vi "field_sweep.vi"() -> ()   [LabVIEW 2017]
uses:
  Controls/State.ctl
  Controls/Data.ctl
  <vilib>/Utility/error.llb/DialogType.ctl
  <vilib>/DAQmx/write.llb/DAQmx Write (Analog DBL 1Chan 1Samp).vi
  <vilib>/DAQmx/create/channels.llb/DAQmx Create Channel (AO-Voltage-Basic).vi
  <vilib>/DAQmx/miscellaneous.llb/DAQmx Fill In Error Info.vi
  <instrlib>/niVNA/niVNA.llb/niVNA Fetch Sweep Measurement (DBL).vi
  <instrlib>/LakeShore 336/Public/Data/Sensor Data (Single Reading).vi
  <instrlib>/LakeShore 336/Lake Shore 336.lvlib
panel:
  in  "Folder":path caption="Folder for saving"
  out "Temp. Cont. Name (out)":refnum<visa-resource-name>
  in  "Temp. Cont. Name (in)":refnum<visa-resource-name>
  in  "Auto Save flag":bool
  out "Gaussmeter Name (out)":refnum<visa-resource-name>="Lakeshore_475"
  in  "Gaussmeter Name (in)":refnum<visa-resource-name>="Lakeshore_475"
  in  "Clear button":bool
  in  "Hysteresis":bool caption="Hysteresis On/Off"
  out "DAQ channel (out)":tag="DAQ_6363/ao1"
  in  "Averaging Points":i32=10 min=1 max=3201 step=1
  in  "DAQ channel (in)":tag="DAQ_6363/ao1"
  in  "Exit Button":bool
  in  "IF Bandwidth":dbl(ring)=1000.0 items=["10 Hz"=10.0, "30 Hz"=30.0, "100 Hz"=100.0, "300 Hz"=300.0, "1 KHz"=1000.0, "3 KHz"=3000.0, "10 KHz"=10000.0, "30 KHz"=30000.0]
  in  "Speed (Oe/sec)":dbl=50.0
  in  "Frequency (Hz)":dbl=3000000000.0 min=10000000.0 max=6000000000.0
  in  "Save Button":bool
  out "Status":string="Off"
  out "Cursor":cluster{"x":dbl, "y":dbl} {"x" format="%.2f"; "y" format="%.5f"}
  out "VNA Name (out)":refnum<k15>="VNA_5630"
  out "Error (out)":errorcluster
  in  "Error (in) (no error)":errorcluster
  in  "Format":i32(ring)=1 items=["Log Magnitude (dB)"=0, "Lin Magnitude"=1, "Phase (deg)"=2, "VSWR"=3, "Group Delay"=6]
  out "SpectrumGraph":cluster{"Old Field":dbl[], "Old Signal":dbl[]}[](graph)
  in  "S-parameter":i32(ring)=1 caption="Measurement" items=["S11", "S21"]
  in  "Start Button":bool
  in  "Stop Button":bool
  in  "Output Power (dBm)":dbl=1.0 min=-25.0 max=5.0 step=0.5
  in  "Number of Points":i32=1000 min=1 max=3201 step=1
  in  "Stop H Field (Oe)":dbl=1500.0 min=-6000.0 max=6000.0 format="%#_6f"
  in  "Start H Field (Oe)":dbl=1000.0 min=-6000.0 max=6000.0 format="%#_6f"
  in  "VNA Name (in)":refnum<k15>="VNA_5630"
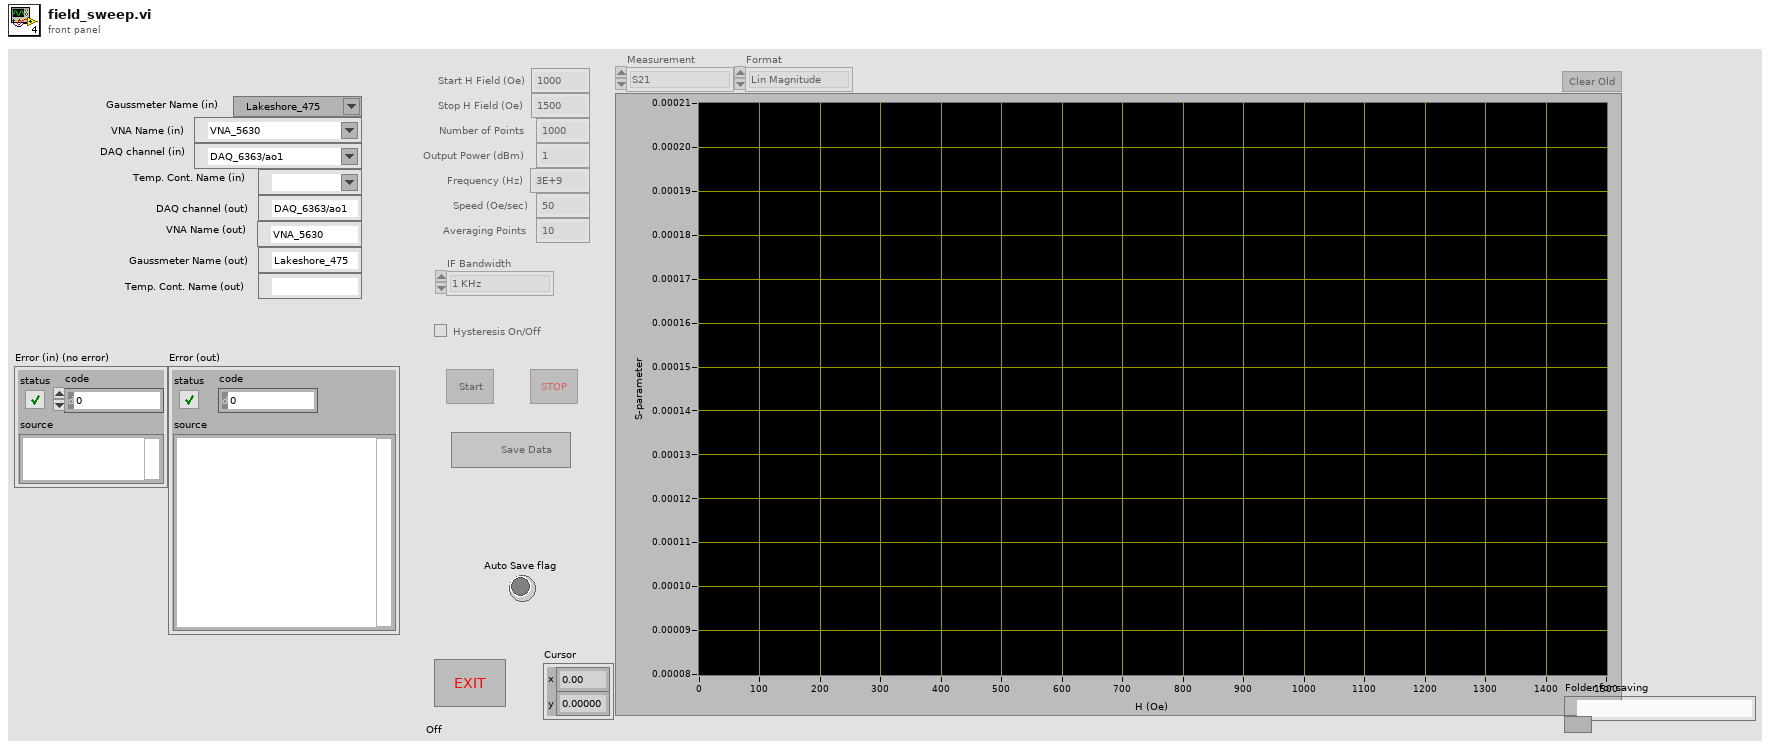
[diagram p1: front panel]
types:
  T1 = cluster{"DAQ task":refnum<k21>, "DAQ channel":tag, "VNA Name":refnum<k15>, "Gaussmeter Name":refnum<visa-resource-name>, "Temp. Cont. Name":refnum<visa-resource-name>}
  T2 = typedef "Data.ctl" = cluster{"Field":dbl[], "Signal":dbl[], "Temperature":dbl[], "Old Field":dbl[], "Old Signal":dbl[], "Old Temperature":dbl[]}
  T3 = typedef "State.ctl" = enum16{"Init", "Idle", "Sweeping up", "Sweeping down", "Running", "Running down", "Shutdown"}
  T4 = cluster{"Baud Rate":u32, "Parity":u16, "Data Bits":u16, "Stop Bits":u16, "Flow Control":u16}
  T5 = typedef "DialogType.ctl" = u16
  T6 = typedef "LVPoint32TypeDef.ctl" = cluster{"Horizontal":i32, "Vertical":i32}
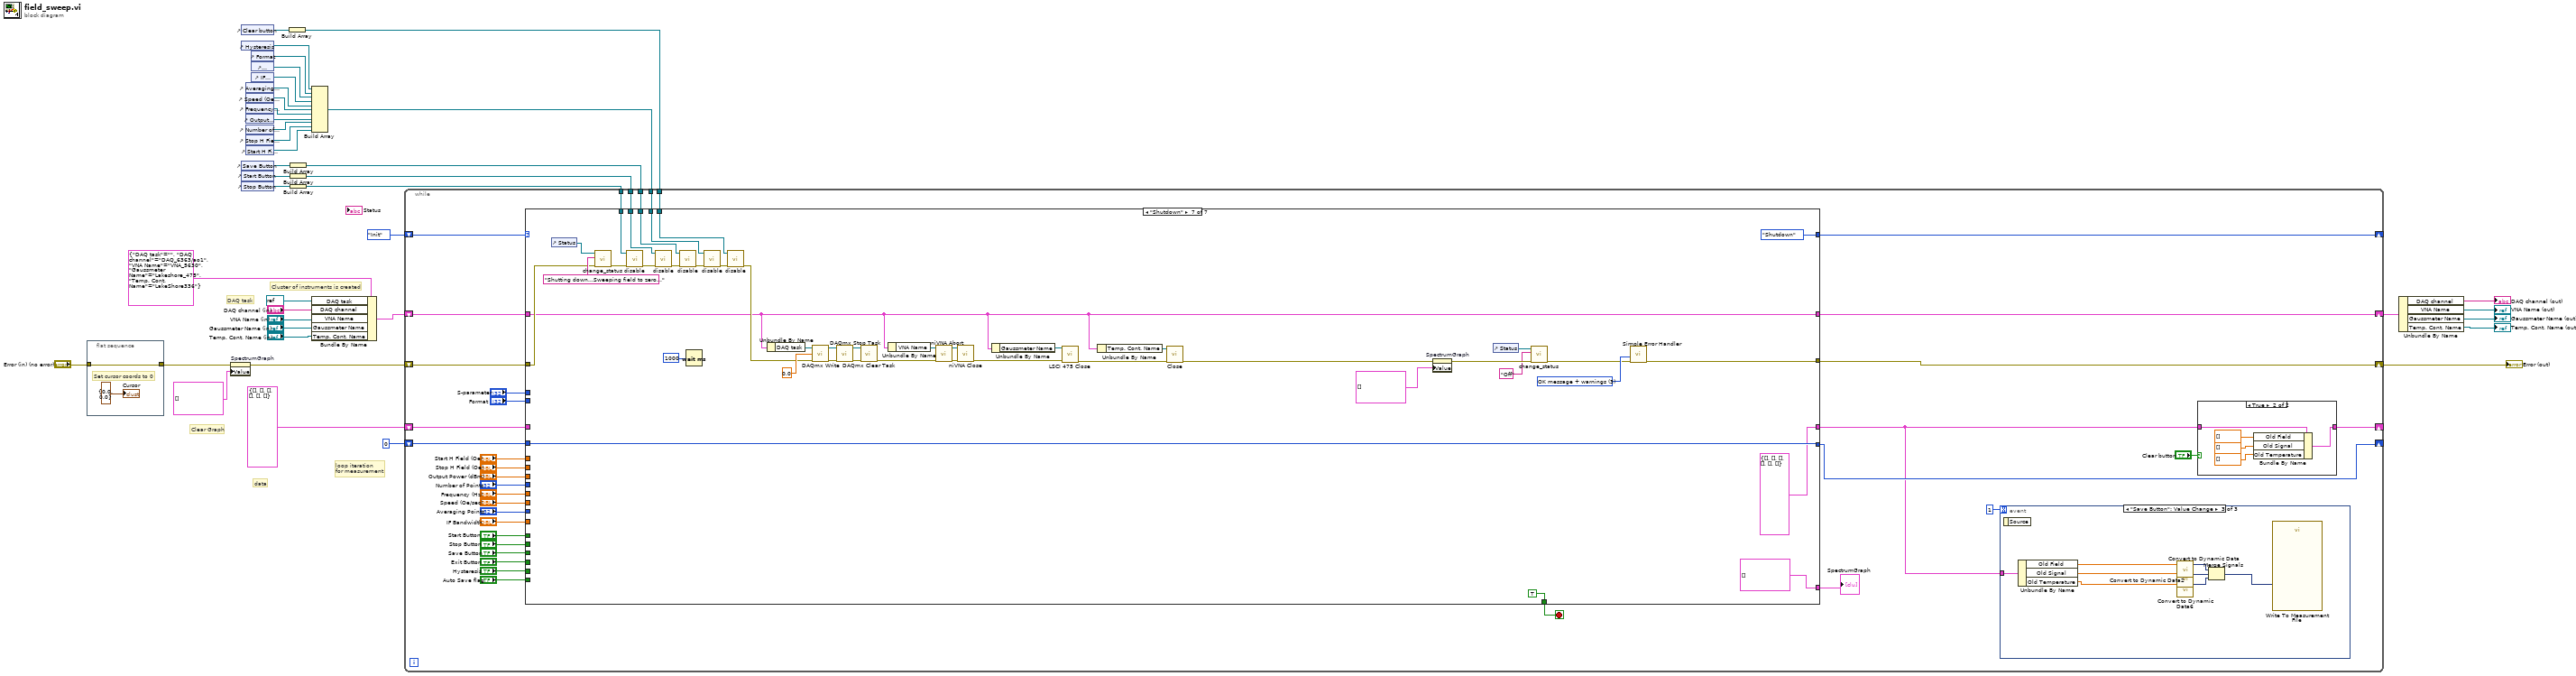
[diagram p0: block diagram]
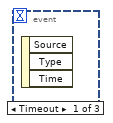
[diagram p3: hidden frame]
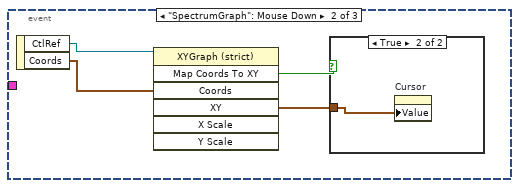
[diagram p4: hidden frame]
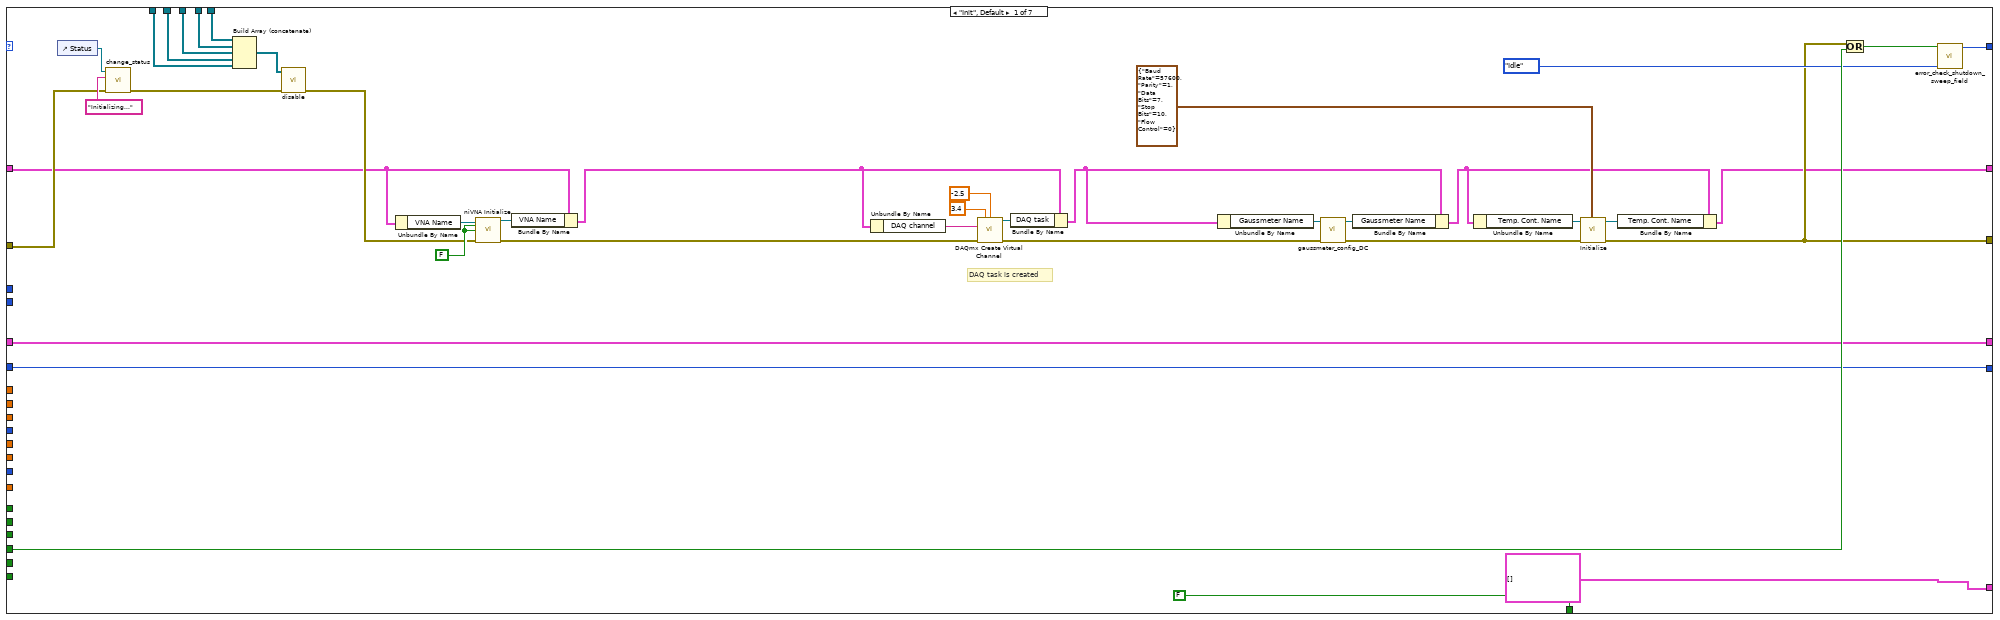
[diagram p6: hidden frame]
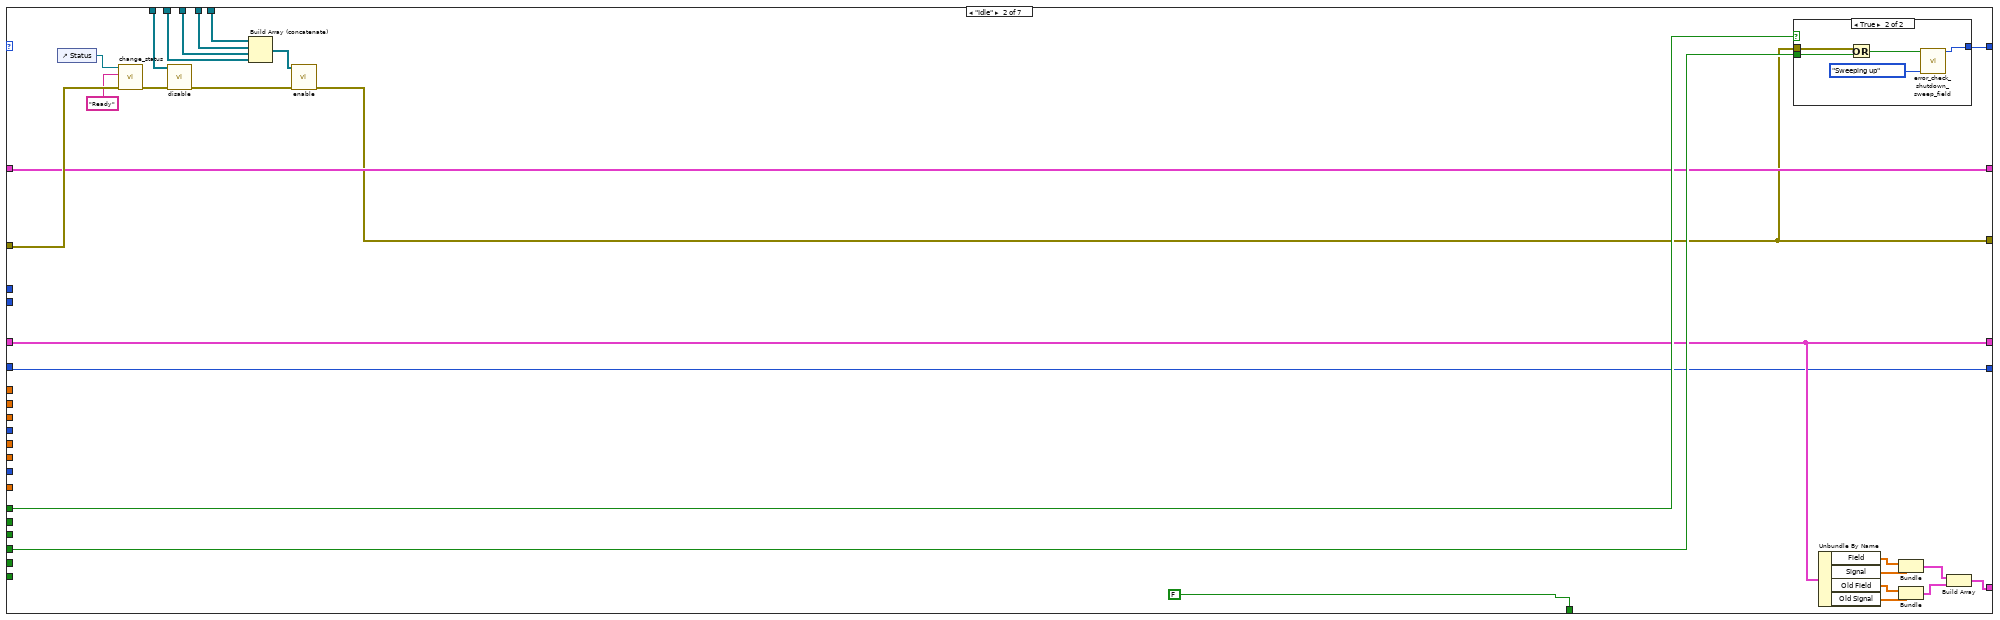
[diagram p7: hidden frame]
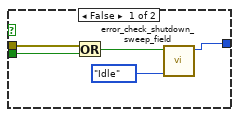
[diagram p8: hidden frame]
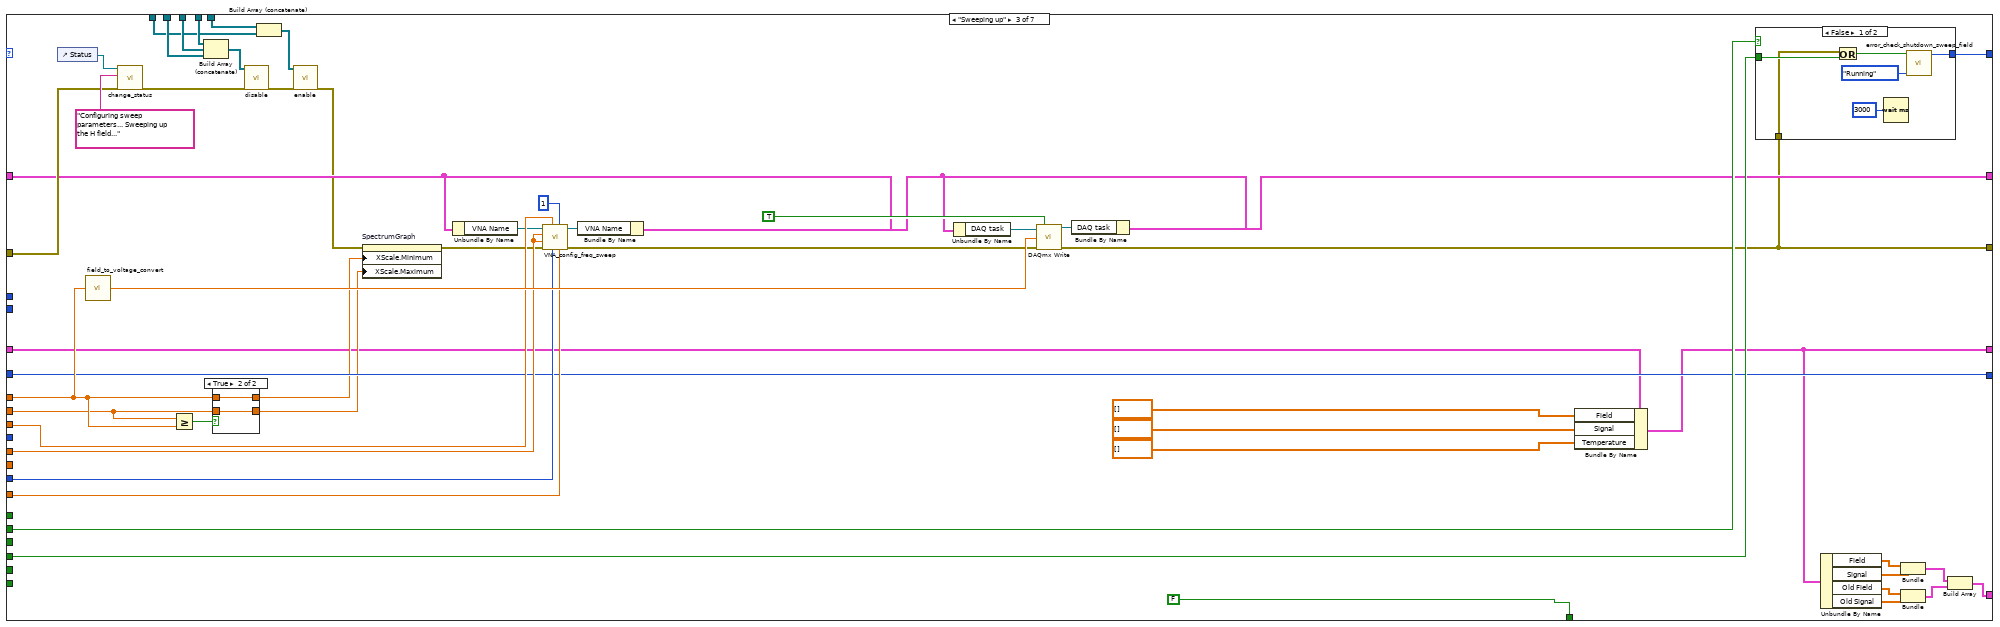
[diagram p9: hidden frame]
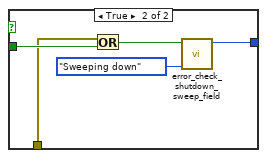
[diagram p11: hidden frame]
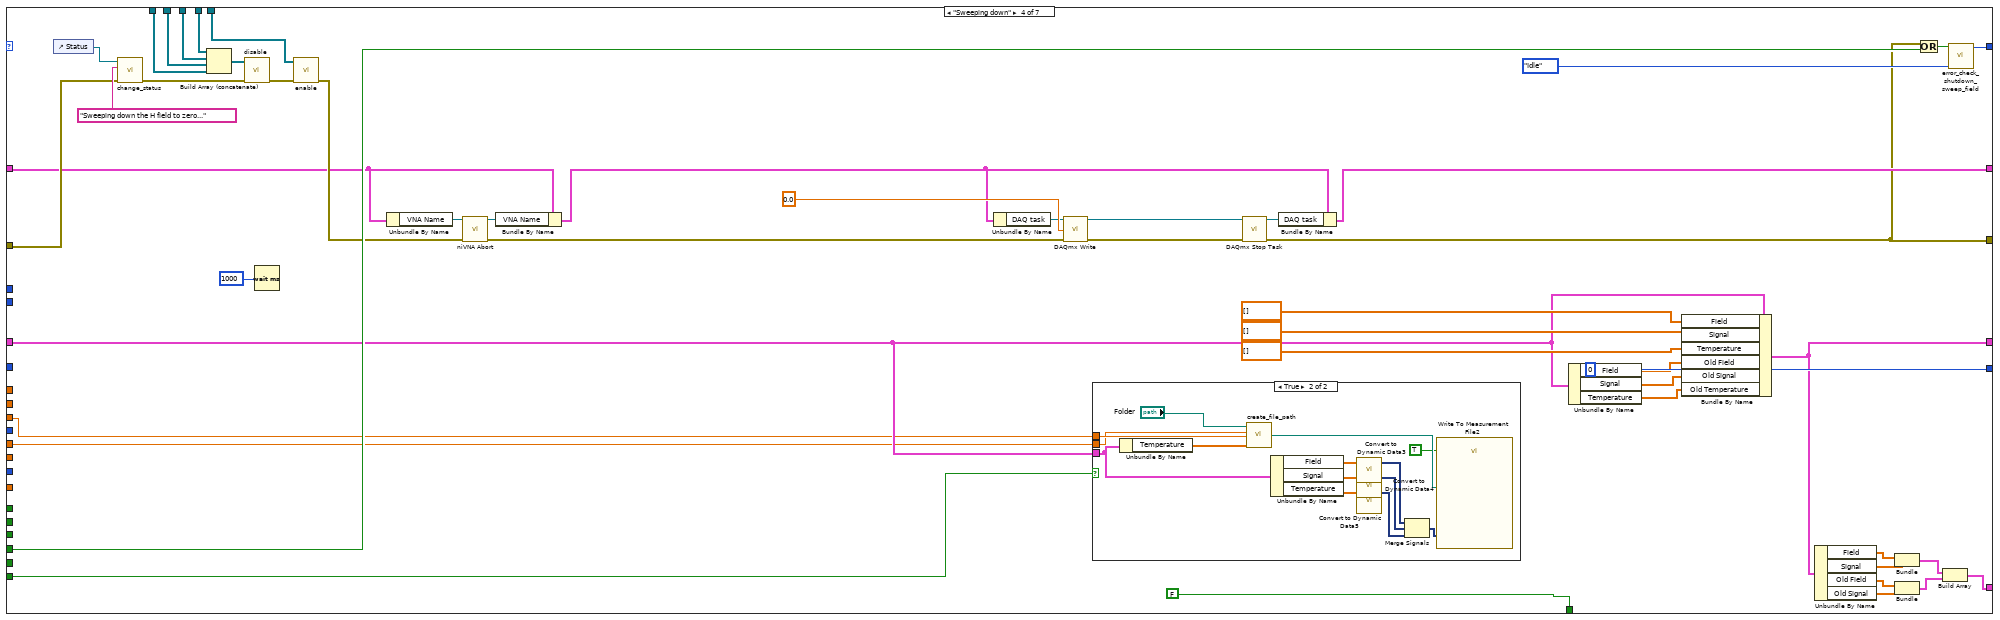
[diagram p12: hidden frame]
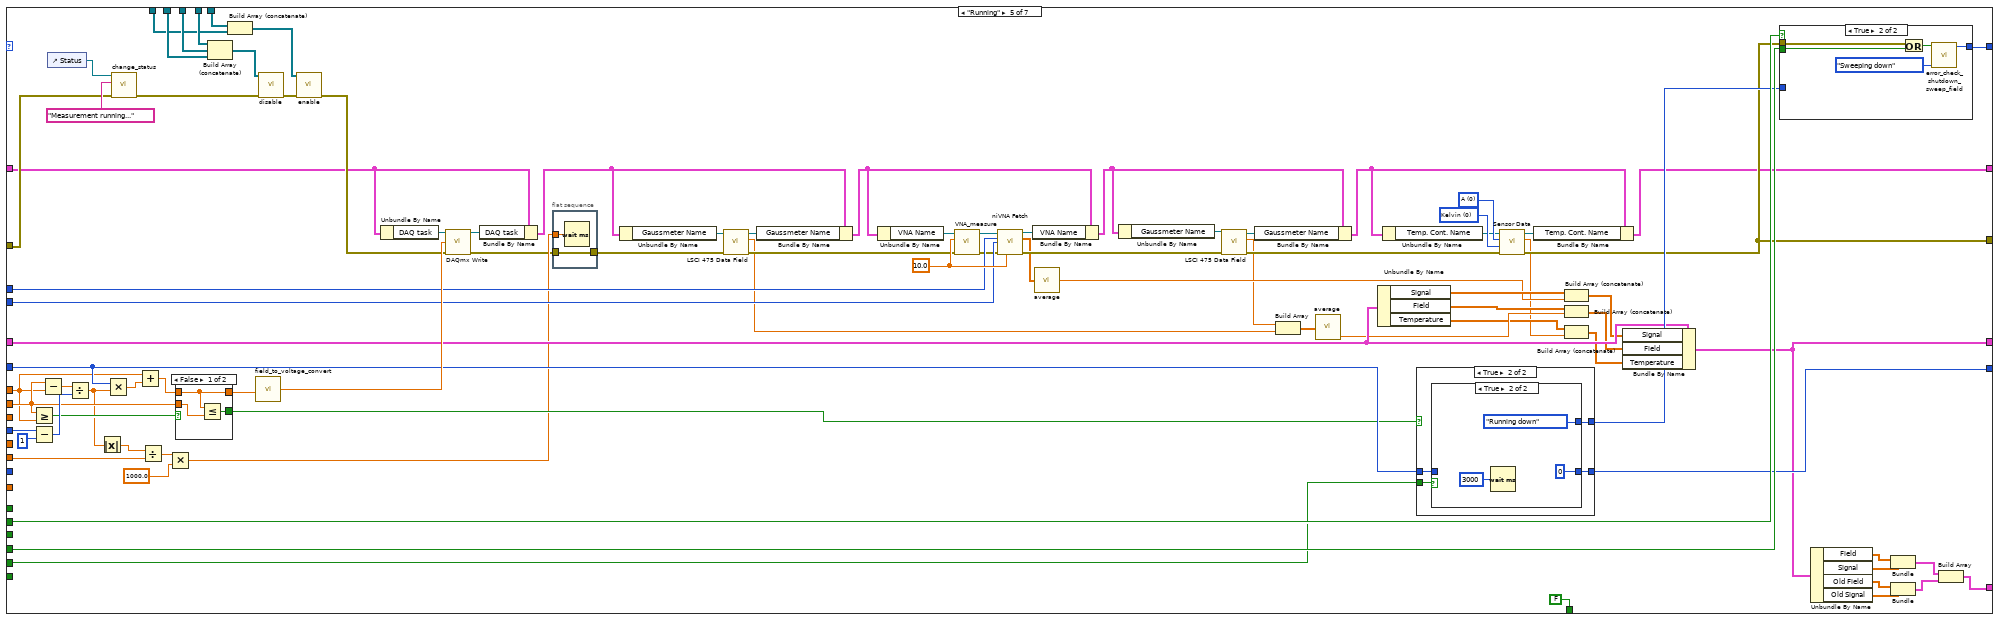
[diagram p14: hidden frame]
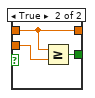
[diagram p15: hidden frame]
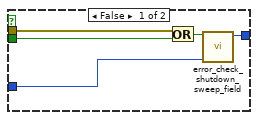
[diagram p16: hidden frame]
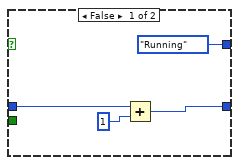
[diagram p17: hidden frame]
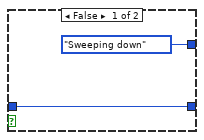
[diagram p18: hidden frame]
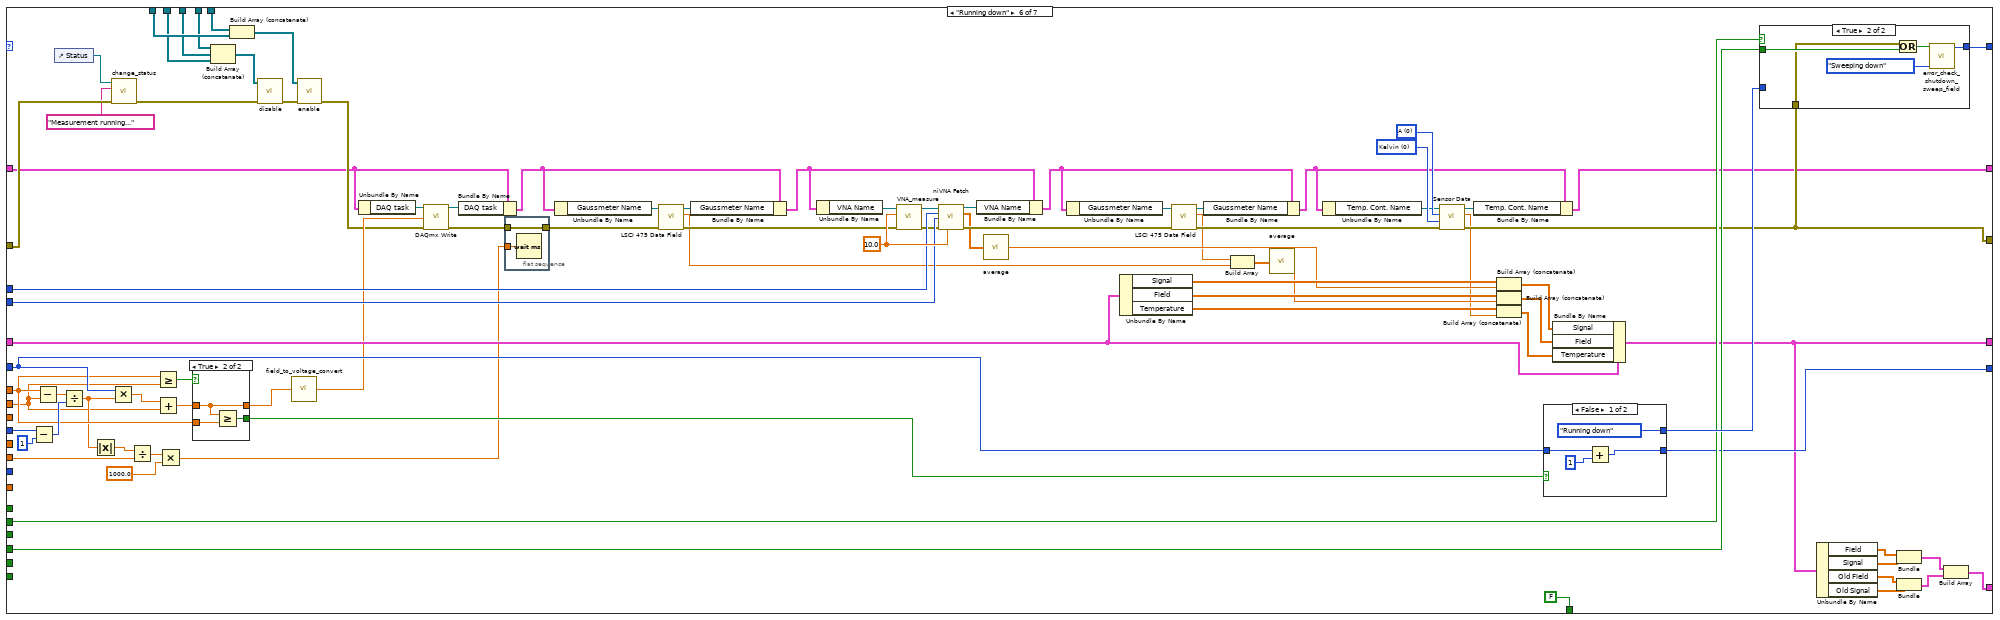
[diagram p19: hidden frame]
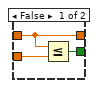
[diagram p20: hidden frame]
diagram:
  # "data"
  # "Cluster of instruments is created"
  # "loop iteration\nfor measurement"
  # "DAQ task"
  # "Clear Graph"
  n1 = flat-sequence {
    tunnel: "Error (in) (no error)" -> [w41]
    tunnel: [w41] -> w7
    frame #0 {
      # "Set cursor coords to 0"
      "Cursor" <- cluster{"x":dbl, "y":dbl} {"x"=0.0, "y"=0.0} ("Cursor")
    }
  }
  n2 = property on="SpectrumGraph" class="XYGraph (strict)"(error in=w7, "Value"=cluster{"Old Field":dbl[], "Old Signal":dbl[]}[] [] ("SpectrumGraph")) -> (error out=w23:errorcluster)  [unwired: 1 in, 1 out]
  n3 = control-ref of="Clear button"() -> (w16:refnum<vi>)
  n4 = control-ref of="Hysteresis"() -> (w17:refnum<vi>)
  n5 = control-ref of="Save Button"() -> (w27:refnum<vi>)
  n6 = control-ref of="Start Button"() -> (w32:refnum<vi>)
  n7 = control-ref of="Stop Button"() -> (w31:refnum<vi>)
  n8 = control-ref of="Averaging Points"() -> (w24:refnum<vi>)
  n9 = control-ref of="Speed (Oe/sec)"() -> (w38:refnum<vi>)
  n10 = control-ref of="Frequency (Hz)"() -> (w37:refnum<vi>)
  n11 = control-ref of="Output Power (dBm)"() -> (w36:refnum<vi>)
  n12 = control-ref of="Number of Points"() -> (w35:refnum<vi>)
  n13 = control-ref of="Stop H Field (Oe)"() -> (w34:refnum<vi>)
  n14 = control-ref of="Start H Field (Oe)"() -> (w33:refnum<vi>)
  n15 = control-ref of="Format"() -> (w18:refnum<vi>)
  n16 = control-ref of="S-parameter"() -> (w19:refnum<vi>)
  n17 = control-ref of="IF Bandwidth"() -> (w39:refnum<vi>)
  n18 = Build Array(w16) -> (w15:refnum<vi>[])
  n19 = Build Array(w27) -> (w26:refnum<vi>[])
  n20 = Build Array(w32) -> (w29:refnum<vi>[])
  n21 = Build Array(w31) -> (w28:refnum<vi>[])
  n22 = Bundle By Name(cluster=T1 {"DAQ task"="", "DAQ channel"="DAQ_6363/ao1", "VNA Name"="VNA_5630", "Gaussmeter Name"="Lakeshore_475", "Temp. Cont. Name"="LakeShore336"} ("Cluster"), "DAQ task"=refnum<k21> refnum ("task in"), "DAQ channel"="DAQ channel (in)", "VNA Name"="VNA Name (in)", "Gaussmeter Name"="Gaussmeter Name (in)", "Temp. Cont. Name"="Temp. Cont. Name (in)") -> (w9:T1)
  n23 = Build Array(w17, w18, w19, w39, w24, w38, w37, w36, w35, w34, w33) -> (w30:refnum<vi>[])
  n24 = while {
    shift-right: [w74] -> _
    shift-left: State."Init" -> [w78]
    shift-right: [w57] -> _
    shift-left: 0 -> [w59]
    tunnel: w30 -> [w77]
    tunnel: w29 -> [w76]
    tunnel: w28 -> [w75]
    shift-right: [w73] -> w20
    shift-left: w23 -> [w72]
    tunnel: w26 -> [w71]
    shift-right: [w48] -> _
    shift-left: T2 {"Field"=[], "Signal"=[], "Temperature"=[], "Old Field"=[], "Old Signal"=[], "Old Temperature"=[]} ("Cluster") -> [w54]
    tunnel: w15 -> [w47]
    shift-right: [w45] -> w6
    shift-left: w9 -> [w46]
    stop <- w66 stop-if-true
    n25 = case shown="\"Shutdown\"" w78 {
      tunnel: w77 -> [w103 w142 w184 w260 w311 w429 w571]
      tunnel: w76 -> [w101 w140 w182 w258 w309 w427 w573]
      tunnel: w75 -> [w100 w163 w179 w257 w306 w430 w574]
      tunnel: w72 -> [w134 w161 w223 w288 w391 w513 w569]
      tunnel: [w129 w157 w220 w284 w376 w493 State."Shutdown"] -> w74
      tunnel: [w110 w144 w189 w261 w322 w441 w544] -> w73
      tunnel: w71 -> [w102 w141 w183 w259 w310 w428 w572]
      tunnel: "Start Button" -> [_ w158 _ _ _ _ _]
      tunnel: "Stop Button" -> [_ _ w222 _ w379 w501 _]
      tunnel: "Save Button" -> [_ _ _ _ _ _ _]
      tunnel: "Exit Button" -> [w130 w156 w219 w285 w378 w494 _]
      tunnel: [FALSE FALSE FALSE FALSE FALSE FALSE TRUE] -> w66
      tunnel: "Start H Field (Oe)" -> [_ _ w210 _ w352 w484 _]
      tunnel: "Stop H Field (Oe)" -> [_ _ w209 _ w364 w472 _]
      tunnel: "Output Power (dBm)" -> [_ _ w217 w242 _ _ _]
      tunnel: "Number of Points" -> [_ _ _ _ w386 w487 _]
      tunnel: "Frequency (Hz)" -> [_ _ w218 w243 _ _ _]
      tunnel: "Speed (Oe/sec)" -> [_ _ _ _ w387 w477 _]
      tunnel: w59 -> [w127 w146 w201 _ w380 w488 w559]
      tunnel: "Averaging Points" -> [_ _ w216 _ _ _ _]
      tunnel: [w127 w146 w201 0 w349 w470 w559] -> w57
      tunnel: "IF Bandwidth" -> [_ _ w214 _ _ _ _]
      tunnel: [w125 w147 w185 w268 w348 w469 T2 {"Field"=[], "Signal"=[], "Temperature"=[], "Old Field"=[], "Old Signal"=[], "Old Temperature"=[]} ("Cluster")] -> w43
      tunnel: w54 -> [w125 w147 w186 w244 w374 w500 _]
      tunnel: "Hysteresis" -> [_ _ _ _ w362 _ _]
      tunnel: "S-parameter" -> [_ _ _ _ w361 w503 _]
      tunnel: "Format" -> [_ _ _ _ w360 w502 _]
      tunnel: [cluster{"Old Field":dbl[], "Old Signal":dbl[]}[] [] w148 w202 w269 w359 w483 cluster{"Old Field":dbl[], "Old Signal":dbl[]}[] []] -> w50
      tunnel: w47 -> [w104 w143 w181 w266 w307 w431 w550]
      tunnel: w46 -> [w118 w145 w198 w250 w344 w465 w539]
      tunnel: [w105 w145 w190 w264 w319 w439 w539] -> w45
      tunnel: "Auto Save flag" -> [_ _ _ w241 _ _ _]
      frame "Init", Default {
        w135 = FALSE ("id query")
        # "DAQ task is created"
        n26 = control-ref of="Status"() -> (w137:refnum<vi>)
        n27 = call "change_status.vi"("error in (no error)"=w134, "String"="Initializing...", "String in"=w137) -> ("error out"=w98:errorcluster)  [unwired: 8 in]
        n28 = Build Array (concatenate)(w104, w103, w102, w101, w100) -> (w99:refnum<vi>[])
        n29 = call "disable.vi"("error in (no error)"=w98, "Array"=w99) -> ("error out"=w122:errorcluster)  [unwired: 9 in]
        n30 = Unbundle By Name(w118) -> ("VNA Name"=w121:refnum<k15>)
        n31 = call <instrlib>:"niVNA Initialize.vi"("resource name"=w121, "id query"=w135, "reset"=w135, "error in"=w122) -> ("instrument handle"=w116:refnum<k15>, "error out"=w133:errorcluster)  [unwired: 10 in]
        n32 = Bundle By Name(cluster=w118, "VNA Name"=w116) -> (w117:T1)
        n33 = Unbundle By Name(w117) -> ("DAQ channel"=w120:tag)
        n34 = call-poly <vilib>:"DAQmx Create Virtual Channel.vi"("maximum value"=3.4, "minimum value"=-2.5, "physical channels"=w120, "error in"=w133) -> ("task out"=w119:refnum<k21>, "error out"=w115:errorcluster)  [unwired: 10 in]
        n35 = Bundle By Name(cluster=w117, "DAQ task"=w119) -> (w112:T1)
        n36 = Unbundle By Name(w112) -> ("Gaussmeter Name"=w114:refnum<visa-resource-name>)
        n37 = call "gaussmeter_config_DC.vi"("error in (no error)"=w115, "VISA Refnum in"=w114) -> ("error out"=w111:errorcluster, "VISA Refnum out"=w113:refnum<visa-resource-name>)  [unwired: 8 in]
        n38 = Bundle By Name(cluster=w112, "Gaussmeter Name"=w113) -> (w106:T1)
        n39 = Unbundle By Name(w106) -> ("Temp. Cont. Name"=w108:refnum<visa-resource-name>)
        n40 = call <instrlib>:"Initialize.vi"("Serial Configuration"=T4 {"Baud Rate"=57600, "Parity"=1, "Data Bits"=7, "Stop Bits"=10, "Flow Control"=0}, "error in (no error)"=w111, "VISA resource name"=w108) -> ("error out"=w110:errorcluster, "VISA resource name out"=w107:refnum<visa-resource-name>)  [unwired: 7 in]
        n41 = Bundle By Name(cluster=w106, "Temp. Cont. Name"=w107) -> (w105:T1)
        n42 = Or(x=w110, y=w130) -> (x .or. y?=w128:bool)
        n43 = call "error_check_shutdown_sweep_field.vi"("State In"=State."Idle", "Boolean"=w128) -> ("State Out"=w129:T3)  [unwired: 9 in]
      }
      frame "Idle" {
        n44 = control-ref of="Status"() -> (w160:refnum<vi>)
        n45 = call "change_status.vi"("error in (no error)"=w161, "String"="Ready", "String in"=w160) -> ("error out"=w162:errorcluster)  [unwired: 8 in]
        n46 = call "disable.vi"("error in (no error)"=w162, "Array"=w163) -> ("error out"=w138:errorcluster)  [unwired: 9 in]
        n47 = Build Array (concatenate)(w143, w142, w141, w140) -> (w139:refnum<vi>[])
        n48 = call "enable.vi"("error in (no error)"=w138, "Array"=w139) -> ("error out"=w144:errorcluster)  [unwired: 9 in]
        n49 = case shown="True" w158 {
          tunnel: [w167 w171] -> w157
          tunnel: w156 -> [w166 w172]
          tunnel: w144 -> [w164 w169]
          frame False {
            n50 = Or(x=w164, y=w166) -> (x .or. y?=w168:bool)
            n51 = call "error_check_shutdown_sweep_field.vi"("State In"=State."Idle", "Boolean"=w168) -> ("State Out"=w167:T3)  [unwired: 9 in]
          }
          frame True {
            n52 = Or(x=w169, y=w172) -> (x .or. y?=w173:bool)
            n53 = call "error_check_shutdown_sweep_field.vi"("State In"=State."Sweeping up", "Boolean"=w173) -> ("State Out"=w171:T3)  [unwired: 9 in]
          }
        }
        n54 = Unbundle By Name(w147) -> ("Field"=w154:dbl[], "Signal"=w153:dbl[], "Old Field"=w152:dbl[], "Old Signal"=w151:dbl[])
        n55 = Bundle("Field"=w154, "Signal"=w153) -> (w150:cluster{"Field":dbl[], "Signal":dbl[]})  [unwired: 1 in]
        n56 = Bundle("Old Field"=w152, "Old Signal"=w151) -> (w149:cluster{"Old Field":dbl[], "Old Signal":dbl[]})  [unwired: 1 in]
        n57 = Build Array(w150, w149) -> (w148:cluster{"Old Field":dbl[], "Old Signal":dbl[]}[])
      }
      frame "Sweeping up" {
        n58 = control-ref of="Status"() -> (w224:refnum<vi>)
        n59 = call "field_to_voltage_convert.vi"("Start H Field (Oe)"=w210) -> ("Numeric"=w221:dbl)
        n60 = call "change_status.vi"("error in (no error)"=w223, "String"="Configuring sweep parameters... Sweeping up the H field...", "String in"=w224) -> ("error out"=w177:errorcluster)  [unwired: 8 in]
        n61 = Greater Or Equal?(x=w209, y=w210) -> (x >= y?=w211:bool)
        n62 = Build Array (concatenate)(w184, w183, w182) -> (w180:refnum<vi>[])
        n63 = case shown="True" w211 {
          tunnel: w210 -> [w227 w229]
          tunnel: w209 -> [w226 w228]
          tunnel: [w226 w229] -> w195
          tunnel: [w227 w228] -> w196
          frame False {
          }
          frame True {
          }
        }
        n64 = call "disable.vi"("error in (no error)"=w177, "Array"=w180) -> ("error out"=w176:errorcluster)  [unwired: 9 in]
        n65 = Build Array (concatenate)(w181, w179) -> (w178:refnum<vi>[])
        n66 = call "enable.vi"("error in (no error)"=w176, "Array"=w178) -> ("error out"=w175:errorcluster)  [unwired: 9 in]
        n67 = property on="SpectrumGraph" class="XYGraph (strict)"(error in=w175, "XScale.Minimum"=w195, "XScale.Maximum"=w196) -> (error out=w200:errorcluster)  [unwired: 1 in, 1 out]
        n68 = Unbundle By Name(w198) -> ("VNA Name"=w199:refnum<k15>)
        n69 = call "VNA_config_freq_sweep.vi"("IF Bandwidth"=w214, "Averaging"=1, "Number of Points"=w216, "Output Power"=w217, "error in (no error)"=w200, "Stop Frequency"=w218, "Start Frequency"=w218, "Resource Name In"=w199) -> ("error out"=w194:errorcluster, "Resource Name Out"=w197:refnum<k15>)  [unwired: 2 in]
        n70 = Bundle By Name(cluster=w198, "VNA Name"=w197) -> (w191:T1)
        n71 = Unbundle By Name(w191) -> ("DAQ task"=w193:refnum<k21>)
        n72 = call-poly <vilib>:"DAQmx Write.vi"("task/channels in"=w193, "auto start"=TRUE, "data"=w221, "error in"=w194) -> ("task out"=w192:refnum<k21>, "error out"=w189:errorcluster)  [unwired: 9 in, 1 out]
        n73 = Bundle By Name(cluster=w191, "DAQ task"=w192) -> (w190:T1)
        n74 = Bundle By Name(cluster=w186, "Field"=dbl[] [], "Signal"=dbl[] [], "Temperature"=dbl[] []) -> (w185:T2)
        n75 = case shown="False" w222 {
          tunnel: [w234 w239] -> w220
          tunnel: w219 -> [w231 w238]
          tunnel: w189 -> [w230 w236]
          frame False {
            n76 = Or(x=w230, y=w231) -> (x .or. y?=w235:bool)
            n77 = Wait (ms)(milliseconds to wait=u32 3000) -> ()  [unwired: 1 out]
            n78 = call "error_check_shutdown_sweep_field.vi"("State In"=State."Running", "Boolean"=w235) -> ("State Out"=w234:T3)  [unwired: 9 in]
          }
          frame True {
            n79 = Or(x=w236, y=w238) -> (x .or. y?=w240:bool)
            n80 = call "error_check_shutdown_sweep_field.vi"("State In"=State."Sweeping down", "Boolean"=w240) -> ("State Out"=w239:T3)  [unwired: 9 in]
          }
        }
        n81 = Unbundle By Name(w185) -> ("Field"=w208:dbl[], "Signal"=w207:dbl[], "Old Field"=w206:dbl[], "Old Signal"=w205:dbl[])
        n82 = Bundle("Field"=w208, "Signal"=w207) -> (w204:cluster{"Field":dbl[], "Signal":dbl[]})  [unwired: 1 in]
        n83 = Bundle("Old Field"=w206, "Old Signal"=w205) -> (w203:cluster{"Old Field":dbl[], "Old Signal":dbl[]})  [unwired: 1 in]
        n84 = Build Array(w204, w203) -> (w202:cluster{"Old Field":dbl[], "Old Signal":dbl[]}[])
      }
      frame "Sweeping down" {
        n85 = control-ref of="Status"() -> (w283:refnum<vi>)
        n86 = call "change_status.vi"("error in (no error)"=w288, "String"="Sweeping down the H field to zero...", "String in"=w283) -> ("error out"=w255:errorcluster)  [unwired: 8 in]
        n87 = Build Array (concatenate)(w260, w259, w258, w257) -> (w256:refnum<vi>[])
        n88 = call "disable.vi"("error in (no error)"=w255, "Array"=w256) -> ("error out"=w267:errorcluster)  [unwired: 9 in]
        n89 = Wait (ms)(milliseconds to wait=u32 1000) -> ()  [unwired: 1 out]
        n90 = call "enable.vi"("error in (no error)"=w267, "Array"=w266) -> ("error out"=w254:errorcluster)  [unwired: 9 in]
        n91 = Unbundle By Name(w250) -> ("VNA Name"=w252:refnum<k15>)
        n92 = call <instrlib>:"niVNA Abort.vi"("instrument handle"=w252, "error in"=w254) -> ("instrument handle out"=w251:refnum<k15>, "error out"=w253:errorcluster)  [unwired: 12 in]
        n93 = Bundle By Name(cluster=w250, "VNA Name"=w251) -> (w249:T1)
        n94 = Unbundle By Name(w249) -> ("DAQ task"=w263:refnum<k21>)
        n95 = call-poly <vilib>:"DAQmx Write.vi"("task/channels in"=w263, "data"=0.0, "error in"=w253) -> ("task out"=w281:refnum<k21>, "error out"=w280:errorcluster)  [unwired: 10 in, 1 out]
        n96 = case shown="True" w241 {
          tunnel: w244 -> [_ w296]
          tunnel: w242 -> [_ w293]
          tunnel: w243 -> [_ w292]
          frame False {
          }
          frame True {
            n97 = Unbundle By Name(w296) -> ("Temperature"=w294:dbl[])
            n98 = call "create_file_path.vi"("Old Temperature"=w294, "Output Power (dBm)"=w293, "Frequency (Hz)"=w292, "Folder"="Folder") -> ("file path"=w295:path)
            n99 = Unbundle By Name(w296) -> ("Field"=w303:dbl[], "Signal"=w301:dbl[], "Temperature"=w297:dbl[])
            n100 = call "Convert to Dynamic Data3"("Array"=w303) -> ("Dynamic Data Type"=w302:dynamicdata)  [unwired: 3 in]
            n101 = call "Convert to Dynamic Data4"("Array"=w301) -> ("Dynamic Data Type"=w300:dynamicdata)  [unwired: 3 in]
            n102 = call "Convert to Dynamic Data5"("Array"=w297) -> ("Dynamic Data Type"=w298:dynamicdata)  [unwired: 3 in]
            n103 = Merge Signals(w302, w300, w298) -> (w299:dynamicdata)
            n104 = call "Write To Measurement File2"("Signals"=w299, "Reset"=TRUE, "Filename"=w295) -> ()  [unwired: 14 in, 3 out]
          }
        }
        n105 = call <vilib>:"DAQmx Stop Task.vi"("task/channels in"=w281, "error in"=w280) -> ("task out"=w265:refnum<k21>, "error out"=w261:errorcluster)  [unwired: 12 in]
        n106 = Bundle By Name(cluster=w249, "DAQ task"=w265) -> (w264:T1)
        n107 = Unbundle By Name(w244) -> ("Field"=w247:dbl[], "Signal"=w246:dbl[], "Temperature"=w245:dbl[])
        n108 = Bundle By Name(cluster=w244, "Field"=dbl[] [], "Signal"=dbl[] [], "Temperature"=dbl[] [], "Old Field"=w247, "Old Signal"=w246, "Old Temperature"=w245) -> (w268:T2)
        n109 = Unbundle By Name(w268) -> ("Field"=w275:dbl[], "Signal"=w274:dbl[], "Old Field"=w273:dbl[], "Old Signal"=w272:dbl[])
        n110 = Bundle("Field"=w275, "Signal"=w274) -> (w271:cluster{"Field":dbl[], "Signal":dbl[]})  [unwired: 1 in]
        n111 = Bundle("Old Field"=w273, "Old Signal"=w272) -> (w270:cluster{"Old Field":dbl[], "Old Signal":dbl[]})  [unwired: 1 in]
        n112 = Or(x=w261, y=w285) -> (x .or. y?=w286:bool)
        n113 = Build Array(w271, w270) -> (w269:cluster{"Old Field":dbl[], "Old Signal":dbl[]}[])
        n114 = call "error_check_shutdown_sweep_field.vi"("State In"=State."Idle", "Boolean"=w286) -> ("State Out"=w284:T3)  [unwired: 9 in]
      }
      frame "Running" {
        w325 = u16 0 items=["Kelvin", "Celsius", "Sensor Units"] ("Data Source (0:Kelvin)")
        w326 = u16 0 items=["A", "B", "C", "D"] ("Input (0:A)")
        w388 = 10.0 ("timeout")
        n115 = Greater Or Equal?(x=w364, y=w352) -> (x >= y?=w365:bool)
        n116 = Subtract(x=w386, y=1) -> (x-y=w389:i32)
        n117 = Subtract(x=w364, y=w352) -> (x-y=w384:dbl)
        n118 = control-ref of="Status"() -> (w392:refnum<vi>)
        n119 = Divide(x=w384, y=w389) -> (x/y=w355:dbl)
        n120 = Absolute Value(x=w355) -> (abs(x)=w354:dbl)
        n121 = Multiply(x=w380, y=w355) -> (x*y=w351:dbl)
        n122 = call "change_status.vi"("error in (no error)"=w391, "String"="Measurement running...", "String in"=w392) -> ("error out"=w304:errorcluster)  [unwired: 8 in]
        n123 = Add(x=w352, y=w351) -> (x+y=w350:dbl)
        n124 = Divide(x=w354, y=w387) -> (x/y=w358:dbl)
        n125 = Multiply(x=w358, y=1000.0) -> (x*y=w356:dbl)
        n126 = case shown="False" w365 {
          tunnel: [w394 w397] -> w381
          tunnel: w364 -> [w396 w398]
          tunnel: [w395 w399] -> w363
          tunnel: w350 -> [w394 w397]
          frame False {
            n127 = Less Or Equal?(x=w394, y=w396) -> (x <= y?=w395:bool)
          }
          frame True {
            n128 = Greater Or Equal?(x=w397, y=w398) -> (x >= y?=w399:bool)
          }
        }
        n129 = Build Array (concatenate)(w311, w310, w309) -> (w308:refnum<vi>[])
        n130 = Build Array (concatenate)(w307, w306) -> (w305:refnum<vi>[])
        n131 = call "field_to_voltage_convert.vi"("Start H Field (Oe)"=w381) -> ("Numeric"=w385:dbl)
        n132 = call "disable.vi"("error in (no error)"=w304, "Array"=w308) -> ("error out"=w353:errorcluster)  [unwired: 9 in]
        n133 = call "enable.vi"("error in (no error)"=w353, "Array"=w305) -> ("error out"=w347:errorcluster)  [unwired: 9 in]
        n134 = Unbundle By Name(w344) -> ("DAQ task"=w346:refnum<k21>)
        n135 = call-poly <vilib>:"DAQmx Write.vi"("task/channels in"=w346, "data"=w385, "error in"=w347) -> ("task out"=w345:refnum<k21>, "error out"=w343:errorcluster)  [unwired: 10 in, 1 out]
        n136 = Bundle By Name(cluster=w344, "DAQ task"=w345) -> (w330:T1)
        n137 = flat-sequence {
          tunnel: w356 -> [w424]
          tunnel: w343 -> [w423]
          tunnel: [w423] -> w332
          frame #0 {
            n138 = Wait (ms)(milliseconds to wait=w424) -> ()  [unwired: 1 out]
          }
        }
        n139 = Unbundle By Name(w330) -> ("Gaussmeter Name"=w334:refnum<visa-resource-name>)
        n140 = call <instrlib>:"LSCI 475 Data Field.vi"("error in (no error)"=w332, "VISA session"=w334) -> ("error out"=w331:errorcluster, "Field Reading"=w315:dbl, "dup VISA session"=w333:refnum<visa-resource-name>)  [unwired: 7 in]
        n141 = Bundle By Name(cluster=w330, "Gaussmeter Name"=w333) -> (w329:T1)
        n142 = Unbundle By Name(w329) -> ("VNA Name"=w342:refnum<k15>)
        n143 = call "VNA_measure.vi"("error in (no error)"=w331, "timeout"=w388, "Resource Name In"=w342) -> ("error out"=w341:errorcluster, "Resource Name Out"=w340:refnum<k15>)  [unwired: 7 in]
        n144 = call-poly <instrlib>:"niVNA Fetch.vi"("instrument handle"=w340, "measurement"=w361, "format"=w360, "error in"=w341, "timeout"=w388) -> ("instrument handle out"=w339:refnum<k15>, "data"=w327:dbl[], "error out"=w338:errorcluster)  [unwired: 7 in, 1 out]
        n145 = Bundle By Name(cluster=w329, "VNA Name"=w339) -> (w335:T1)
        n146 = call "average.vi"("Array"=w327) -> ("Average"=w328:dbl)
        n147 = Unbundle By Name(w335) -> ("Gaussmeter Name"=w337:refnum<visa-resource-name>)
        n148 = call <instrlib>:"LSCI 475 Data Field.vi"("error in (no error)"=w338, "VISA session"=w337) -> ("error out"=w323:errorcluster, "Field Reading"=w317:dbl, "dup VISA session"=w336:refnum<visa-resource-name>)  [unwired: 7 in]
        n149 = Bundle By Name(cluster=w335, "Gaussmeter Name"=w336) -> (w320:T1)
        n150 = Build Array(w317, w315) -> (w318:dbl[])
        n151 = call "average.vi"("Array"=w318) -> ("Average"=w316:dbl)
        n152 = Unbundle By Name(w374) -> ("Signal"=w383:dbl[], "Field"=w382:dbl[], "Temperature"=w313:dbl[])
        n153 = Unbundle By Name(w320) -> ("Temp. Cont. Name"=w324:refnum<visa-resource-name>)
        n154 = case shown="True" w363 {
          tunnel: [State."Running" w417] -> w377
          tunnel: w380 -> [w412 w416]
          tunnel: [w410 w414] -> w349
          tunnel: w362 -> [_ w415]
          frame False {
            n155 = Add(x=w412, y=1) -> (x+y=w410:i32)
          }
          frame True {
            n156 = case shown="True" w415 {
              tunnel: [State."Sweeping down" State."Running down"] -> w417
              tunnel: w416 -> [w418 _]
              tunnel: [w418 0] -> w414
              frame False {
              }
              frame True {
                n157 = Wait (ms)(milliseconds to wait=u32 3000) -> ()  [unwired: 1 out]
              }
            }
          }
        }
        n158 = call-poly <instrlib>:"Sensor Data.vi"("error in (no error)"=w323, "Data Source (0:Kelvin)"=w325, "Input (0:A)"=w326, "VISA resource name"=w324) -> ("error out"=w322:errorcluster, "Sensor Data"=w312:dbl, "VISA resource name out"=w321:refnum<visa-resource-name>)  [unwired: 5 in]
        n159 = Bundle By Name(cluster=w320, "Temp. Cont. Name"=w321) -> (w319:T1)
        n160 = Build Array (concatenate)(w383, w328) -> (w373:dbl[])
        n161 = Build Array (concatenate)(w382, w316) -> (w372:dbl[])
        n162 = Build Array (concatenate)(w313, w312) -> (w314:dbl[])
        n163 = Bundle By Name(cluster=w374, "Signal"=w373, "Field"=w372, "Temperature"=w314) -> (w348:T2)
        n164 = case shown="True" w379 {
          tunnel: [w403 w408] -> w376
          tunnel: w378 -> [w402 w407]
          tunnel: w377 -> [w401 _]
          tunnel: w322 -> [w400 w405]
          frame False {
            n165 = Or(x=w400, y=w402) -> (x .or. y?=w404:bool)
            n166 = call "error_check_shutdown_sweep_field.vi"("State In"=w401, "Boolean"=w404) -> ("State Out"=w403:T3)  [unwired: 9 in]
          }
          frame True {
            n167 = Or(x=w405, y=w407) -> (x .or. y?=w409:bool)
            n168 = call "error_check_shutdown_sweep_field.vi"("State In"=State."Sweeping down", "Boolean"=w409) -> ("State Out"=w408:T3)  [unwired: 9 in]
          }
        }
        n169 = Unbundle By Name(w348) -> ("Field"=w371:dbl[], "Signal"=w370:dbl[], "Old Field"=w369:dbl[], "Old Signal"=w368:dbl[])
        n170 = Bundle("Field"=w371, "Signal"=w370) -> (w367:cluster{"Field":dbl[], "Signal":dbl[]})  [unwired: 1 in]
        n171 = Bundle("Old Field"=w369, "Old Signal"=w368) -> (w366:cluster{"Old Field":dbl[], "Old Signal":dbl[]})  [unwired: 1 in]
        n172 = Build Array(w367, w366) -> (w359:cluster{"Old Field":dbl[], "Old Signal":dbl[]}[])
      }
      frame "Running down" {
        w445 = u16 0 items=["Kelvin", "Celsius", "Sensor Units"] ("Data Source (0:Kelvin)")
        w446 = u16 0 items=["A", "B", "C", "D"] ("Input (0:A)")
        w510 = 10.0 ("timeout")
        n173 = Subtract(x=w487, y=1) -> (x-y=w491:i32)
        n174 = Subtract(x=w484, y=w472) -> (x-y=w490:dbl)
        n175 = control-ref of="Status"() -> (w512:refnum<vi>)
        n176 = Divide(x=w490, y=w491) -> (x/y=w476:dbl)
        n177 = Absolute Value(x=w476) -> (abs(x)=w475:dbl)
        n178 = Multiply(x=w488, y=w476) -> (x*y=w473:dbl)
        n179 = call "change_status.vi"("error in (no error)"=w513, "String"="Measurement running...", "String in"=w512) -> ("error out"=w432:errorcluster)  [unwired: 8 in]
        n180 = Divide(x=w475, y=w477) -> (x/y=w480:dbl)
        n181 = Greater Or Equal?(x=w484, y=w472) -> (x >= y?=w489:bool)
        n182 = Add(x=w473, y=w472) -> (x+y=w471:dbl)
        n183 = Multiply(x=w480, y=1000.0) -> (x*y=w478:dbl)
        n184 = case shown="True" w489 {
          tunnel: [w514 w517] -> w485
          tunnel: [w516 w519] -> w486
          tunnel: w484 -> [w515 w518]
          tunnel: w471 -> [w514 w517]
          frame False {
            n185 = Less Or Equal?(x=w514, y=w515) -> (x <= y?=w516:bool)
          }
          frame True {
            n186 = Greater Or Equal?(x=w517, y=w518) -> (x >= y?=w519:bool)
          }
        }
        n187 = Build Array (concatenate)(w429, w428, w427) -> (w425:refnum<vi>[])
        n188 = Build Array (concatenate)(w431, w430) -> (w426:refnum<vi>[])
        n189 = call "disable.vi"("error in (no error)"=w432, "Array"=w425) -> ("error out"=w474:errorcluster)  [unwired: 9 in]
        n190 = call "field_to_voltage_convert.vi"("Start H Field (Oe)"=w485) -> ("Numeric"=w482:dbl)
        n191 = call "enable.vi"("error in (no error)"=w474, "Array"=w426) -> ("error out"=w468:errorcluster)  [unwired: 9 in]
        n192 = Unbundle By Name(w465) -> ("DAQ task"=w467:refnum<k21>)
        n193 = call-poly <vilib>:"DAQmx Write.vi"("task/channels in"=w467, "data"=w482, "error in"=w468) -> ("task out"=w466:refnum<k21>, "error out"=w460:errorcluster)  [unwired: 10 in, 1 out]
        n194 = Bundle By Name(cluster=w465, "DAQ task"=w466) -> (w451:T1)
        n195 = flat-sequence {
          tunnel: w478 -> [w537]
          tunnel: w460 -> [w536]
          tunnel: [w536] -> w453
          frame #0 {
            n196 = Wait (ms)(milliseconds to wait=w537) -> ()  [unwired: 1 out]
          }
        }
        n197 = Unbundle By Name(w451) -> ("Gaussmeter Name"=w455:refnum<visa-resource-name>)
        n198 = call <instrlib>:"LSCI 475 Data Field.vi"("error in (no error)"=w453, "VISA session"=w455) -> ("error out"=w452:errorcluster, "Field Reading"=w437:dbl, "dup VISA session"=w454:refnum<visa-resource-name>)  [unwired: 7 in]
        n199 = Bundle By Name(cluster=w451, "Gaussmeter Name"=w454) -> (w450:T1)
        n200 = Unbundle By Name(w450) -> ("VNA Name"=w464:refnum<k15>)
        n201 = call "VNA_measure.vi"("error in (no error)"=w452, "timeout"=w510, "Resource Name In"=w464) -> ("error out"=w463:errorcluster, "Resource Name Out"=w462:refnum<k15>)  [unwired: 7 in]
        n202 = call-poly <instrlib>:"niVNA Fetch.vi"("instrument handle"=w462, "measurement"=w503, "format"=w502, "error in"=w463, "timeout"=w510) -> ("instrument handle out"=w461:refnum<k15>, "data"=w449:dbl[], "error out"=w457:errorcluster)  [unwired: 7 in, 1 out]
        n203 = Bundle By Name(cluster=w450, "VNA Name"=w461) -> (w456:T1)
        n204 = call "average.vi"("Array"=w449) -> ("Average"=w448:dbl)
        n205 = Unbundle By Name(w456) -> ("Gaussmeter Name"=w459:refnum<visa-resource-name>)
        n206 = Unbundle By Name(w500) -> ("Signal"=w509:dbl[], "Field"=w508:dbl[], "Temperature"=w447:dbl[])
        n207 = call <instrlib>:"LSCI 475 Data Field.vi"("error in (no error)"=w457, "VISA session"=w459) -> ("error out"=w442:errorcluster, "Field Reading"=w438:dbl, "dup VISA session"=w458:refnum<visa-resource-name>)  [unwired: 7 in]
        n208 = Bundle By Name(cluster=w456, "Gaussmeter Name"=w458) -> (w440:T1)
        n209 = Build Array(w438, w437) -> (w436:dbl[])
        n210 = call "average.vi"("Array"=w436) -> ("Average"=w435:dbl)
        n211 = Unbundle By Name(w440) -> ("Temp. Cont. Name"=w444:refnum<visa-resource-name>)
        n212 = call-poly <instrlib>:"Sensor Data.vi"("error in (no error)"=w442, "Data Source (0:Kelvin)"=w445, "Input (0:A)"=w446, "VISA resource name"=w444) -> ("error out"=w441:errorcluster, "Sensor Data"=w433:dbl, "VISA resource name out"=w443:refnum<visa-resource-name>)  [unwired: 5 in]
        n213 = Bundle By Name(cluster=w440, "Temp. Cont. Name"=w443) -> (w439:T1)
        n214 = Build Array (concatenate)(w509, w448) -> (w506:dbl[])
        n215 = Build Array (concatenate)(w508, w435) -> (w505:dbl[])
        n216 = Build Array (concatenate)(w447, w433) -> (w434:dbl[])
        n217 = case shown="False" w486 {
          tunnel: [State."Running down" State."Sweeping down"] -> w507
          tunnel: w488 -> [w532 w534]
          tunnel: [w530 w534] -> w470
          frame False {
            n218 = Add(x=w532, y=1) -> (x+y=w530:i32)
          }
          frame True {
          }
        }
        n219 = Bundle By Name(cluster=w500, "Signal"=w506, "Field"=w505, "Temperature"=w434) -> (w469:T2)
        n220 = case shown="True" w501 {
          tunnel: [w523 w528] -> w493
          tunnel: w494 -> [w522 w527]
          tunnel: w507 -> [w521 _]
          tunnel: w441 -> [w520 w525]
          frame False {
            n221 = Or(x=w520, y=w522) -> (x .or. y?=w524:bool)
            n222 = call "error_check_shutdown_sweep_field.vi"("State In"=w521, "Boolean"=w524) -> ("State Out"=w523:T3)  [unwired: 9 in]
          }
          frame True {
            n223 = Or(x=w525, y=w527) -> (x .or. y?=w529:bool)
            n224 = call "error_check_shutdown_sweep_field.vi"("State In"=State."Sweeping down", "Boolean"=w529) -> ("State Out"=w528:T3)  [unwired: 9 in]
          }
        }
        n225 = Unbundle By Name(w469) -> ("Field"=w495:dbl[], "Signal"=w496:dbl[], "Old Field"=w497:dbl[], "Old Signal"=w498:dbl[])
        n226 = Bundle("Field"=w495, "Signal"=w496) -> (w504:cluster{"Field":dbl[], "Signal":dbl[]})  [unwired: 1 in]
        n227 = Bundle("Old Field"=w497, "Old Signal"=w498) -> (w499:cluster{"Old Field":dbl[], "Old Signal":dbl[]})  [unwired: 1 in]
        n228 = Build Array(w504, w499) -> (w483:cluster{"Old Field":dbl[], "Old Signal":dbl[]}[])
      }
      frame "Shutdown" {
        w565 = T5 3 items=["no dialog", "OK message", "continue or stop message", "OK message + warnings", "continue/stop + warnings"] ("type of dialog (OK msg:1)")
        n229 = control-ref of="Status"() -> (w570:refnum<vi>)
        n230 = call "change_status.vi"("error in (no error)"=w569, "String"="Shutting down...Sweeping field to zero...", "String in"=w570) -> ("error out"=w576:errorcluster)  [unwired: 8 in]
        n231 = call "disable.vi"("error in (no error)"=w576, "Array"=w574) -> ("error out"=w579:errorcluster)  [unwired: 9 in]
        n232 = call "disable.vi"("error in (no error)"=w579, "Array"=w573) -> ("error out"=w578:errorcluster)  [unwired: 9 in]
        n233 = call "disable.vi"("error in (no error)"=w578, "Array"=w572) -> ("error out"=w577:errorcluster)  [unwired: 9 in]
        n234 = Wait (ms)(milliseconds to wait=u32 1000) -> ()  [unwired: 1 out]
        n235 = call "disable.vi"("error in (no error)"=w577, "Array"=w571) -> ("error out"=w551:errorcluster)  [unwired: 9 in]
        n236 = call "disable.vi"("error in (no error)"=w551, "Array"=w550) -> ("error out"=w549:errorcluster)  [unwired: 9 in]
        n237 = Unbundle By Name(w539) -> ("DAQ task"=w548:refnum<k21>)
        n238 = call-poly <vilib>:"DAQmx Write.vi"("task/channels in"=w548, "data"=0.0, "error in"=w549) -> ("task out"=w561:refnum<k21>, "error out"=w562:errorcluster)  [unwired: 10 in, 1 out]
        n239 = call <vilib>:"DAQmx Stop Task.vi"("task/channels in"=w561, "error in"=w562) -> ("task out"=w566:refnum<k21>, "error out"=w567:errorcluster)  [unwired: 12 in]
        n240 = call <vilib>:"DAQmx Clear Task.vi"("task in"=w566, "error in"=w567) -> ("error out"=w560:errorcluster)  [unwired: 13 in]
        n241 = Unbundle By Name(w539) -> ("VNA Name"=w547:refnum<k15>)
        n242 = call <instrlib>:"niVNA Abort.vi"("instrument handle"=w547, "error in"=w560) -> ("instrument handle out"=w546:refnum<k15>, "error out"=w568:errorcluster)  [unwired: 12 in]
        n243 = call <instrlib>:"niVNA Close.vi"("instrument handle"=w546, "error in"=w568) -> ("error out"=w543:errorcluster)  [unwired: 13 in]
        n244 = Unbundle By Name(w539) -> ("Gaussmeter Name"=w542:refnum<visa-resource-name>)
        n245 = call <instrlib>:"LSCI 475 Close.vi"("VISA session"=w542, "error in (no error)"=w543) -> ("error out"=w541:errorcluster)  [unwired: 13 in]
        n246 = Unbundle By Name(w539) -> ("Temp. Cont. Name"=w540:refnum<visa-resource-name>)
        n247 = call <instrlib>:"Close.vi"("error in (no error)"=w541, "VISA resource name"=w540) -> ("error out"=w538:errorcluster)  [unwired: 9 in]
        n248 = property on="SpectrumGraph" class="XYGraph (strict)"(error in=w538, "Value"=cluster{"Old Field":dbl[], "Old Signal":dbl[]}[] [] ("SpectrumGraph")) -> (error out=w556:errorcluster)  [unwired: 1 in, 1 out]
        n249 = control-ref of="Status"() -> (w553:refnum<vi>)
        n250 = call "change_status.vi"("error in (no error)"=w556, "String"="Off", "String in"=w553) -> ("error out"=w555:errorcluster)  [unwired: 8 in]
        n251 = call <vilib>:"Simple Error Handler.vi"("type of dialog (OK msg:1)"=w565, "error in (no error)"=w555) -> ("error out"=w544:errorcluster)  [unwired: 3 in, 4 out]
      }
    }
    "SpectrumGraph" <- w50
    n252 = event shown="[2] \"Save Button\": Value Change" {
      selector: _ -> [_ _ _]
      dyn-events: _ -> [_ _ _]
      timeout: 1 -> [_ _ _]
      tunnel: w43 -> [_ _ w97]
      event Timeout {
        n253 = event-data() -> ()  [unwired: 1 in, 3 out]
      }
      event "SpectrumGraph": Mouse Down {
        n254 = event-data() -> ("CtlRef"=w86:refnum<vi>, "Coords"=w85:T6)  [unwired: 1 in]
        n255 = invoke on="Invoke Node" class="XYGraph (strict)" method="Map Coords To XY"(reference=w86, "Coords"=w85) -> ("Map Coords To XY"=w87:bool, "XY"=w88:cluster{"X":dbl, "Y":dbl})  [unwired: 5 in, 5 out]
        n256 = case shown="True" w87 {
          tunnel: w88 -> [_ w89]
          frame False {
          }
          frame True {
            n257 = property on="Cursor" class="Clust (strict)"("Value"=w89) -> ()  [unwired: 2 in, 2 out]
          }
        }
      }
      event "Save Button": Value Change {
        n258 = event-data() -> ()  [unwired: 1 in, 1 out]
        n259 = Unbundle By Name(w97) -> ("Old Field"=w96:dbl[], "Old Signal"=w93:dbl[], "Old Temperature"=w91:dbl[])
        n260 = call "Convert to Dynamic Data"("Array"=w96) -> ("Dynamic Data Type"=w95:dynamicdata)  [unwired: 3 in]
        n261 = call "Convert to Dynamic Data2"("Array"=w93) -> ("Dynamic Data Type"=w92:dynamicdata)  [unwired: 3 in]
        n262 = call "Convert to Dynamic Data6"("Array"=w91) -> ("Dynamic Data Type"=w90:dynamicdata)  [unwired: 3 in]
        n263 = Merge Signals(w95, w92, w90) -> (w94:dynamicdata)
        n264 = call "Write To Measurement File"("Signals"=w94) -> ()  [unwired: 16 in, 3 out]
      }
    }
    n265 = case shown="True" "Clear button" {
      tunnel: w43 -> [w79 w84]
      tunnel: [w79 w83] -> w48
      frame False {
      }
      frame True {
        n266 = Bundle By Name(cluster=w84, "Old Field"=dbl[] [], "Old Signal"=dbl[] [], "Old Temperature"=dbl[] []) -> (w83:T2)
      }
    }
  }
  "Error (out)" <- w20
  n267 = Unbundle By Name(w6) -> ("DAQ channel"=→"DAQ channel (out)":tag, "VNA Name"=→"VNA Name (out)":refnum<k15>, "Gaussmeter Name"=→"Gaussmeter Name (out)":refnum<visa-resource-name>, "Temp. Cont. Name"=→"Temp. Cont. Name (out)":refnum<visa-resource-name>)
